vi "Test Export Strings.vi"(4 "error in":errorcluster) -> (0 "error out":errorcluster)   [LabVIEW 2025]
doc: "Unit Test for <i>Export Strings.vi</i>. This test generates all VIs, Clusters, Classes and Projects according to the respective definition files, exports the strings with the VI-under-test, and checks that all strings from the definition file are present in the output file."
uses:
  <vilib>/addons/_JKI Toolkits/Caraya/classes/Assert/Assert False.vi
  <vilib>/regexp/Match Regular Expression.xnode
  <vilib>/addons/_JKI Toolkits/Caraya/classes/Test/Test.lvclass
  <vilib>/addons/_JKI Toolkits/Caraya/classes/Assert/Assert.lvclass
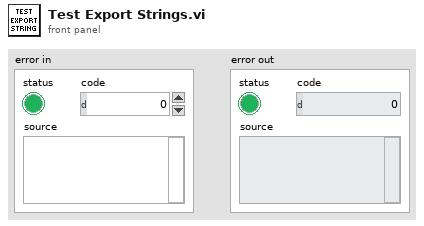
[diagram p1: front panel]
types:
  T1 = typedef "Element Strings--cluster.ctl" = cluster{"Element Name":string, "Strings":string[]}
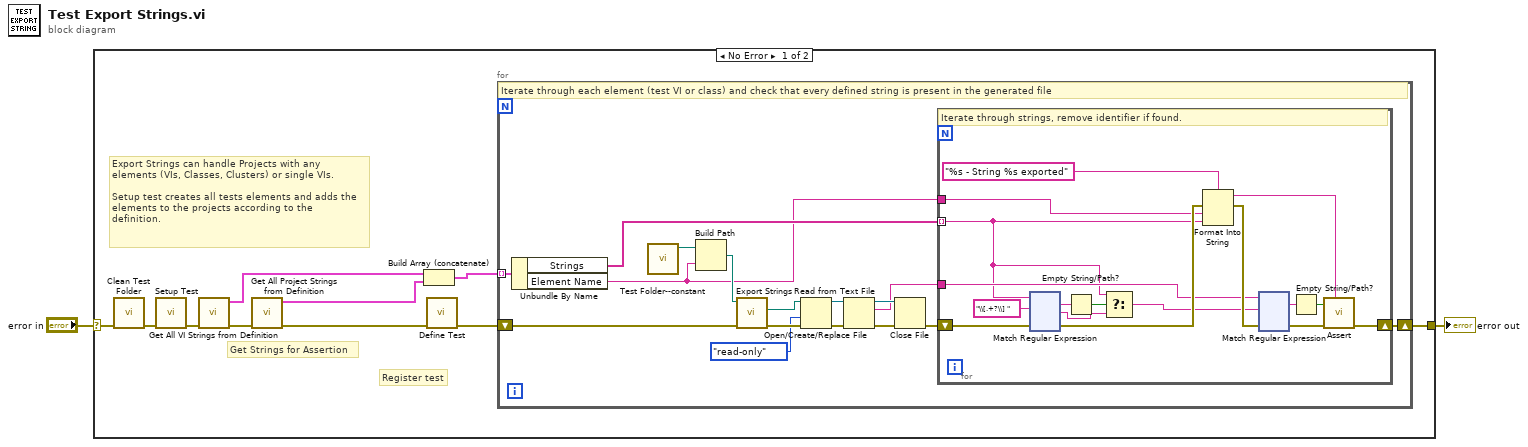
[diagram p0: block diagram]
diagram:
  n1 = case shown="No Error" "error in" {
    selector: "error in" -> [w8 w280]
    tunnel: [w7 w280] -> w2
    frame No Error {
      # "Export Strings can handle Projects with any\nelements (VIs, Classes, Clusters) or single VIs.\n\nSetup test creates all tests elements and adds the\nelements to the projects according to the\ndefinition."
      # "Register test"
      # "Get Strings for Assertion"
      n2 = call "Clean Test Folder.vi"("error in"=w8) -> ("error out"=w12:errorcluster)  [unwired: 6 in]
      n3 = call "Setup Test.vi"("error in"=w12) -> ("error out"=w6:errorcluster)  [unwired: 6 in]
      n4 = call "Get All VI Strings from Definition.vi"("error in"=w6) -> ("error out"=w11:errorcluster, "VI Strings"=w4:T1[])  [unwired: 5 in]
      n5 = call "Get All Project Strings from Definition.vi"("error in"=w11) -> ("error out"=w10:errorcluster, "Project Strings"=w3:T1[])  [unwired: 5 in]
      n6 = Build Array (concatenate)(w4, w3) -> (w5:T1[])
      n7 = call <vilib>:"Define Test.vi"("error in (no error)"=w10) -> ("error out"=w9:errorcluster)  [unwired: 9 in, 1 out]
      n8 = for {
        tunnel: w5 -> [w22] mode=indexing
        shift-right: [w24] -> w7
        shift-left: w9 -> [w28]
        # "Iterate through each element (test VI or class) and check that every defined string is present in the generated file"
        n9 = Unbundle By Name(w22) -> ("Strings"=w15:string[], "Element Name"=w13:string)
        n10 = call "Test Folder--constant.vi"() -> ("Test Folder"=w21:path)  [unwired: 7 in]
        n11 = Build Path(base path=w21, name or relative path=w13) -> (appended path=w20:path)
        n12 = call "Export Strings.vi"("error in"=w28, "Target"=w20) -> ("error out"=w23:errorcluster, "String File Out"=w19:path)  [unwired: 3 in, 1 out]
        n13 = Open/Create/Replace File(file path (use dialog)=w19, error in=w23, access (0:read/write)=enum16{"read/write", "read-only", "write-only"}."read-only") -> (refnum out=w17:refnum<file>, error out=w27:errorcluster)  [unwired: 3 in, 1 out]
        n14 = Read from Text File(file (use dialog)=w17, error in=w27) -> (refnum out=w16:refnum<file>, text=w14:string, error out=w26:errorcluster)  [unwired: 2 in, 1 out]
        n15 = Close File(refnum=w16, error in=w26) -> (error out=w25:errorcluster)  [unwired: 1 out]
        n16 = for {
          tunnel: w15 -> [w31] mode=indexing
          tunnel: w14 -> [w40]
          shift-right: [w44] -> w24
          shift-left: w25 -> [w42]
          tunnel: w13 -> [w35]
          # "Iterate through strings, remove identifier if found."
          n17 = xnode ("Match Regular Expression")("input string"=w31, "regular expression"="\\[.+?\\] ", "error in"=w42) -> ("whole match"=w33:string, "after match"=w30:string, "error out"=w41:errorcluster)  [unwired: 3 in, 2 out]
          n18 = Empty String/Path?(string/path=w33) -> (empty?=w32:bool)
          n19 = Select(t=w31, s=w32, f=w30) -> (s? t:f=w29:string)
          n20 = Format Into String(format string="%s - String %s exported", error in=w41, w35, w31) -> (resulting string=w36:string, error out=w43:errorcluster)  [unwired: 1 in]
          n21 = xnode ("Match Regular Expression")("input string"=w40, "regular expression"=w29, "error in"=w43) -> ("whole match"=w39:string, "error out"=w45:errorcluster)  [unwired: 3 in, 3 out]
          n22 = Empty String/Path?(string/path=w39) -> (empty?=w37:bool)
          n23 = call-poly <vilib>:"Assert.vi"("Label"=w36, "error in (no error)"=w45, "False?"=w37) -> ("error out"=w44:errorcluster)  [unwired: 7 in, 1 out]
        }
      }
    }
    frame Error {
      # "Pass error without further action"
    }
  }
  "error out" <- w2
